vi "FolderMon Archive TDMS.vi"() -> ()   [LabVIEW 2011]
uses:
  <vilib>/Utility/miscctls.llb/LVDateTimeRec.ctl
  DIAdem/lib/DIAdem Daemon Queue.ctl
  DIAdem/lib/DIAdem Daemon Script Type.ctl
  ITK EXT/utils/strutil.llb/Case Matching.ctl
  server lib/Spartan Version.vi
  server lib/Spartan CONFIG Global.vi
  Summitek EXT/OpenG EXT/file/file.llb/File Exists - Scalar__ogtk.vi
  Summitek EXT/OpenG EXT/file/file.llb/Convert File Extension (Path)__ogtk.vi
panel:
  out "Files Archived":i32
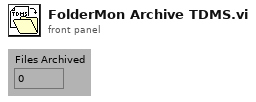
[diagram p1: front panel]
types:
  T1 = typedef "LVDateTimeRec.ctl" = cluster{"fractional second":dbl, "second":i32, "minute":i32, "hour":i32, "day of month":i32, "month":i32, "year":i32, "day of week":i32, "day of year":i32, "DST":i32}
  T2 = typedef "DIAdem Daemon Queue.ctl" = cluster{"Report Template TDM":path, "Report Processor VBS":path, "Report Path PDF":path, "Report Script Params":string, "Username":string, "Script Type":T3, "Report Query Params":string, "Client Machine":string, "Print on Client?":bool, "Response Queue Name":string, "Script Variables":string[], "Start Request Time":timestamp, "Wait?":bool}
  T3 = typedef "DIAdem Daemon Script Type.ctl" = enum16{"Report", "Query", "Script", "Datasheet", "Append", "Restart", "Stop"}
  T4 = typedef "Case Matching.ctl" = enum16{"a != A", "a == A", "system"}
  T5 = typedef "Keyed Array.ctl" = cluster{"keys":string[], "values":string[]}
  T6 = enum16{"open", "open or create", "create or replace", "create", "open (read-only)"}
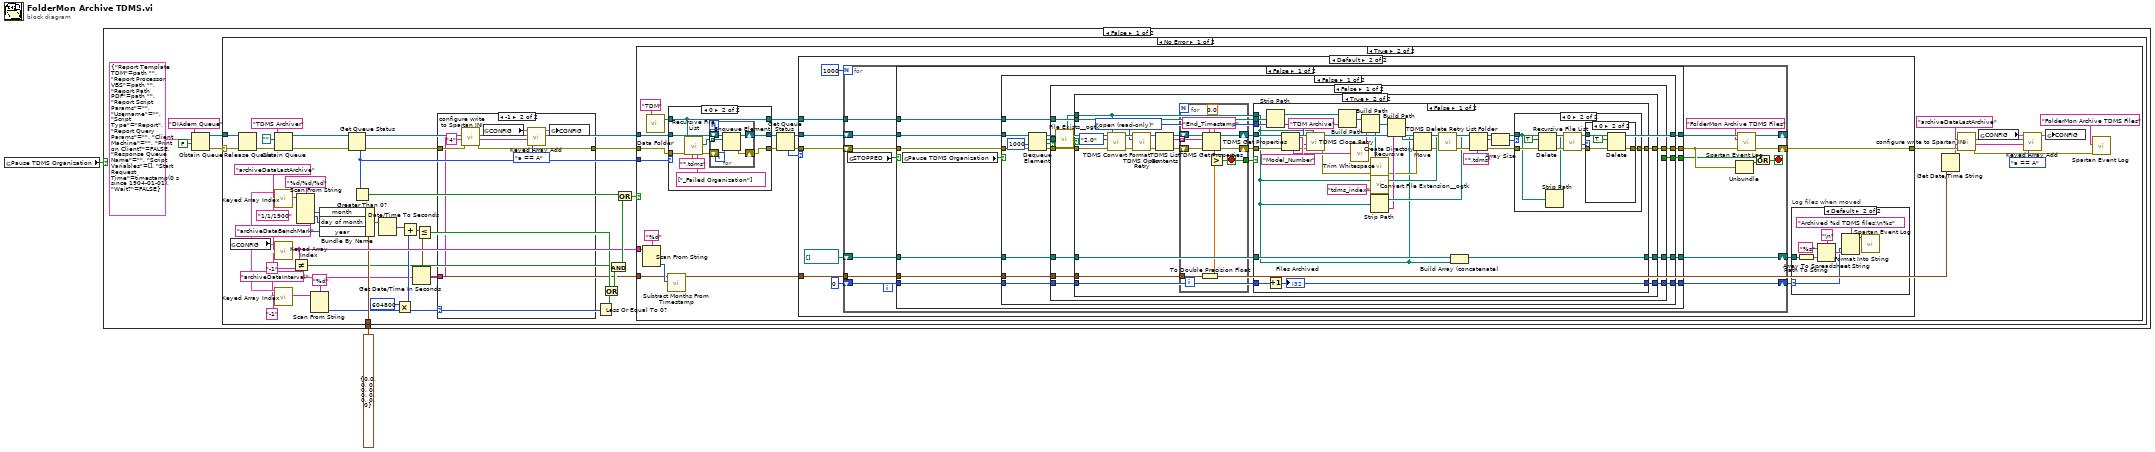
[diagram p0: block diagram]
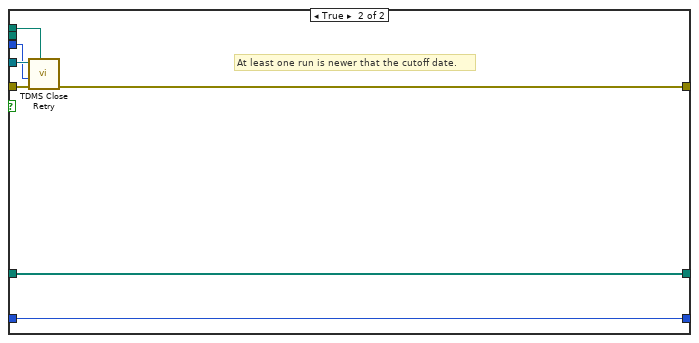
[diagram p9: hidden frame]
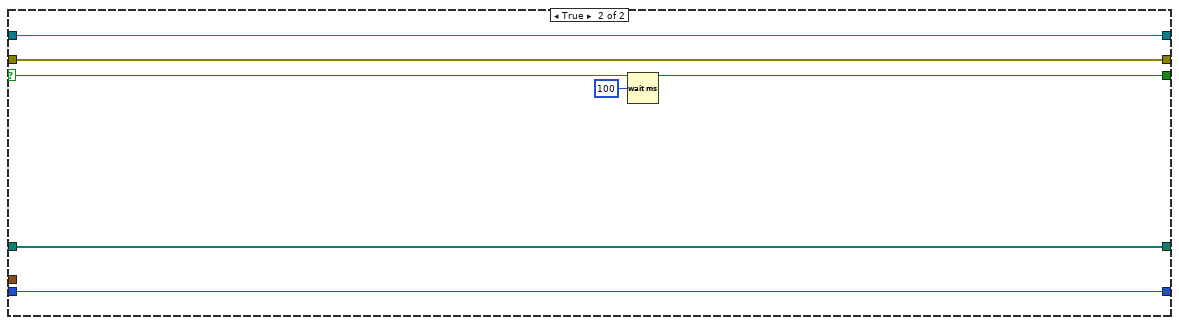
[diagram p11: hidden frame]
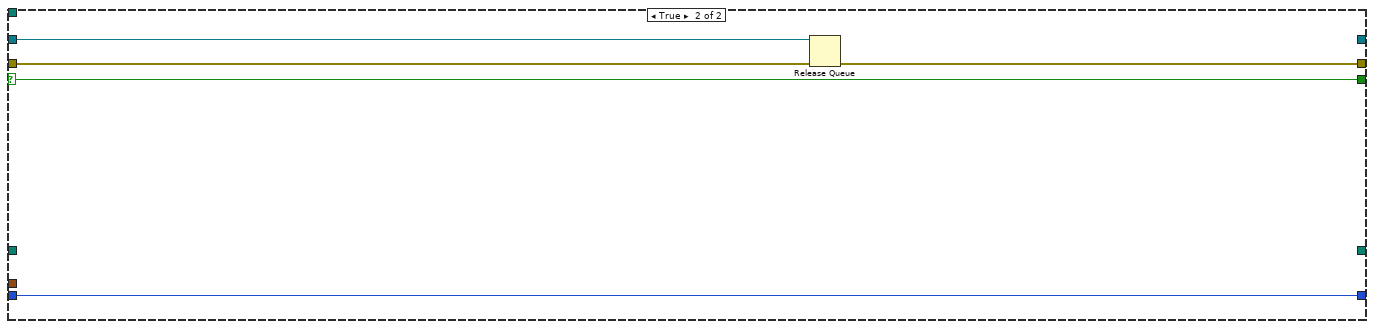
[diagram p12: hidden frame]
diagram:
  n1 = global read "Spartan Version.vi" "Pause TDMS Organization"() -> (w2:bool)
  n2 = case shown="False" w2 {
    tunnel: T1 {"fractional second"=0.0, "second"=0, "minute"=0, "hour"=0, "day of month"=0, "month"=0, "year"=0, "day of week"=0, "day of year"=0, "DST"=0} ("date time rec") -> [w3 _]
    frame False {
      n3 = Obtain Queue(name (unnamed)="DIAdem Queue", element data type=T2 {"Report Template TDM"=path "", "Report Processor VBS"=path "", "Report Path PDF"=path "", "Report Script Params"="", "Username"="", "Script Type"=enum."Report", "Report Query Params"="", "Client Machine"="", "Print on Client?"=FALSE, "Response Queue Name"="", "Script Variables"=[], "Start Request Time"=timestamp(0 s since 1904-01-01), "Wait?"=FALSE} ("DD_Report"), create if not found? (T)=FALSE) -> (queue out=w5:refnum<queue>, error out=w6:errorcluster)  [unwired: 2 in, 1 out]
      n4 = case shown="No Error" w6 {
        selector: w6 -> [w47 _]
        tunnel: w5 -> [w45 _]
        tunnel: w3 -> [w28 _]
        frame No Error {
          w14 = "archiveDataInterval"
          w43 = "-1" ("default value")
          n5 = global read "Spartan CONFIG Global.vi" "CONFIG"() -> (w29:T5)
          n6 = Release Queue(queue=w45, error in (no error)=w47) -> (error out=w46:errorcluster)  [unwired: 1 in, 2 out]
          n7 = Obtain Queue(name (unnamed)="TDMS Archiver", element data type=path "", error in (no error)=w46) -> (queue out=w37:refnum<queue>, error out=w36:errorcluster)  [unwired: 2 in, 1 out]
          n8 = call "Keyed Array Index.vi"("default value"="1/1/1900", "key"="archiveDataLastArchive", "array in"=w29) -> ("value"=w39:string)  [unwired: 1 in, 3 out]
          n9 = call "Keyed Array Index.vi"("default value"=w43, "key"="archiveDataBenchMark", "array in"=w29) -> ("value"=w32:string)  [unwired: 1 in, 3 out]
          n10 = call "Keyed Array Index.vi"("default value"="-1", "key"=w14, "array in"=w29) -> ("value"=w20:string)  [unwired: 1 in, 3 out]
          n11 = Not Equal?(x=w32, y=w43) -> (x != y?=w11:bool)
          n12 = Scan From String(format string="%d/%d/%d", input string=w39) -> (output 1=w27:i32, output 2=w26:i32, output 3=w25:i32)  [unwired: 5 in, 3 out]
          n13 = Scan From String(format string="%d", input string=w20) -> (output 1=w17:i32)  [unwired: 3 in, 3 out]
          n14 = Bundle By Name(cluster=w28, "month"=w27, "day of month"=w26, "year"=w25) -> (w24:T1)
          n15 = Get Queue Status(queue=w37, error in (no error)=w36) -> (queue out=w35:refnum<queue>, error out=w16:errorcluster, # elements in queue=w31:i32)  [unwired: 1 in, 5 out]
          n16 = Greater Than 0?(x=w31) -> (x > 0?=w34:bool)
          n17 = Date/Time To Seconds(2:w24) -> (0:w23:timestamp)  [unwired: 1 in]
          n18 = Multiply(x=604800, y=w17) -> (x*y=w22:i32)
          n19 = Add(x=w23, y=w22) -> (x+y=w18:timestamp)
          n20 = Get Date/Time In Seconds() -> (seconds since 1Jan1904=w9:timestamp)
          n21 = Less Or Equal?(x=w18, y=w9) -> (x <= y?=w13:bool)
          n22 = case shown="-1" w17 {
            tunnel: w16 -> [w50 w53]
            tunnel: [w50 w52] -> w15
            tunnel: w14 -> [_ w51]
            frame Default {
            }
            frame -1 {
              w57 = "4" ("Value (\"\")")
              n23 = call "configure write to Spartan INI.vi"("error in (no error)"=w53, "Value (\"\")"=w57, "Key (\"\")"=w51) -> ("error out"=w52:errorcluster)  [unwired: 8 in]
              n24 = global read "Spartan CONFIG Global.vi" "CONFIG"() -> (w55:T5)
              n25 = call "Keyed Array Add.vi"("case matching (sensitive)"=Case_Matching."a == A", "value"=w57, "key"=w51, "array in"=w55) -> ("array out"=w56:T5)  [unwired: 3 out]
              n26 = global write "Spartan CONFIG Global.vi" "CONFIG"(w56) -> ()
            }
          }
          n27 = Less Or Equal To 0?(x=w17) -> (x <= 0?=w12:bool)
          n28 = Or(x=w13, y=w12) -> (x .or. y?=w10:bool)
          n29 = And(x=w11, y=w10) -> (x .and. y?=w38:bool)
          n30 = Or(x=w34, y=w38) -> (x .or. y?=w33:bool)
          n31 = case shown="True" w33 {
            tunnel: w35 -> [_ w68]
            tunnel: w15 -> [_ w67]
            tunnel: w32 -> [_ w70]
            tunnel: w31 -> [_ w69]
            tunnel: w9 -> [_ w59]
            frame False {
            }
            frame True {
              w61 = "archiveDataLastArchive"
              n32 = Scan From String(format string="%d", input string=w70) -> (output 1=w72:i32)  [unwired: 3 in, 3 out]
              n33 = call "Data Folder.vi"("Relative Path (\"\" - Folder)"="TDM" ("Relative Path (\"\" - Folder)")) -> ("Data Folder"=w78:path)  [unwired: 2 in]
              n34 = call "Subtract Months From Timestamp.vi"("Months"=w72, "Start Time"=w59) -> ("End Time"=w71:timestamp)  [unwired: 9 in]
              n35 = case shown="0" w69 {
                tunnel: w68 -> [w82 w92]
                tunnel: [w84 w87] -> w77
                tunnel: w78 -> [w84 w87]
                tunnel: [w83 w89] -> w79
                tunnel: w67 -> [w83 w93]
                tunnel: [w82 w91] -> w80
                frame Default {
                }
                frame 0 {
                  n36 = call <vilib>:"Recursive File List.vi"("Folders to Exclude"=string[] ["_Failed Organization"], "pattern"="*.tdms", "error in (no error)"=w93, "Folder Path"=w87) -> ("error out"=w90:errorcluster, "All Files in Dir"=w86:path[])  [unwired: 3 in, 3 out]
                  n37 = for {
                    shift-right: [w97] -> w89
                    shift-left: w90 -> [w98]
                    tunnel: w86 -> [w95] mode=indexing
                    shift-right: [w94] -> w91
                    shift-left: w92 -> [w96]
                    n38 = Enqueue Element(queue=w96, element=w95, error in (no error)=w98) -> (queue out=w94:refnum<queue>, error out=w97:errorcluster)  [unwired: 1 in, 1 out]
                  }
                }
              }
              n39 = Get Queue Status(queue=w80, error in (no error)=w79) -> (queue out=w76:refnum<queue>, error out=w75:errorcluster, # elements in queue=w74:i32)  [unwired: 1 in, 5 out]
              n40 = case shown="Default" w74 {
                tunnel: w76 -> [_ w107]
                tunnel: w77 -> [_ w108]
                tunnel: w75 -> [w99 w106]
                tunnel: w71 -> [_ w103]
                tunnel: [w99 w100] -> w63
                frame 0 {
                }
                frame Default {
                  n41 = for {
                    N: 1000 -> [_]
                    tunnel: w108 -> [w122]
                    shift-right: [w115] -> w100
                    shift-left: w106 -> [w125]
                    shift-right: [w123] -> _
                    shift-left: w107 -> [w124]
                    shift-right: [w121] -> w101
                    shift-left: path[] [] -> [w118]
                    shift-right: [w117] -> w102
                    shift-left: 0 -> [w116]
                    tunnel: w103 -> [w114]
                    stop <- w120 stop-if-true
                    n42 = global read "Spartan Version.vi" "STOPPED"() -> (w110:bool)
                    n43 = case shown="False" w110 {
                      selector: w110 -> [_ w262]
                      tunnel: w125 -> [w134 w266]
                      tunnel: w124 -> [w133 w264]
                      tunnel: [w132 _] -> w123
                      tunnel: w122 -> [w137 _]
                      tunnel: [w136 w265] -> w112
                      tunnel: [w135 _] -> w121
                      tunnel: w118 -> [w131 _]
                      tunnel: [w130 w263] -> w117
                      tunnel: w116 -> [w129 w263]
                      tunnel: w114 -> [w127 _]
                      tunnel: [w126 w262] -> w111
                      frame False {
                        n44 = global read "Spartan Version.vi" "Pause TDMS Organization"() -> (w128:bool)
                        n45 = case shown="False" w128 {
                          selector: w128 -> [_ w256]
                          tunnel: w137 -> [w152 _]
                          tunnel: [w151 w261] -> w136
                          tunnel: [w150 w258] -> w135
                          tunnel: w134 -> [w149 w261]
                          tunnel: w133 -> [w147 w260]
                          tunnel: [w146 w260] -> w132
                          tunnel: w131 -> [w142 w258]
                          tunnel: [w141 w259] -> w130
                          tunnel: w129 -> [w140 w259]
                          tunnel: w127 -> [w139 _]
                          tunnel: [w138 w256] -> w126
                          frame False {
                            n46 = Dequeue Element(queue=w147, timeout in ms (-1)=1000, error in (no error)=w149) -> (queue out=w146:refnum<queue>, element=w145:path, timed out?=w143:bool, error out=w148:errorcluster)
                            n47 = case shown="False" w143 {
                              selector: w143 -> [_ w253]
                              tunnel: w152 -> [w162 _]
                              tunnel: [w161 w255] -> w151
                              tunnel: [w158 _] -> w150
                              tunnel: w148 -> [w160 w255]
                              tunnel: w145 -> [w153 _]
                              tunnel: w142 -> [w159 _]
                              tunnel: [w157 w254] -> w141
                              tunnel: w140 -> [w154 w254]
                              tunnel: w139 -> [w155 _]
                              tunnel: [_ w253] -> w138
                              frame False {
                                n48 = call-poly "File Exists__ogtk.vi"("file path"=w153) -> ("exists"=w156:bool)  [unwired: 6 in, 1 out]
                                n49 = case shown="True" w156 {
                                tunnel: w162 -> [_ w170]
                                tunnel: [w165 w172] -> w161
                                tunnel: w160 -> [w165 w185]
                                tunnel: w159 -> [w164 w169]
                                tunnel: [w164 w168] -> w158
                                tunnel: [w163 w166] -> w157
                                tunnel: w153 -> [_ w173]
                                tunnel: w155 -> [_ w177]
                                tunnel: w154 -> [w163 w167]
                                frame False {
                                }
                                frame True {
                                w174 = T6."open (read-only)" ("operation (0:open)")
                                n50 = call <vilib>:"TDMS Convert Format.vi"("error in (no error)"=w185, "target version"=enum16{"1.0", "2.0"}."2.0", "file path"=w173) -> ("error out"=w184:errorcluster, "file path out"=w183:path)  [unwired: 3 in]
                                n51 = call "TDMS Open Retry.vi"("error in (no error)"=w184, "Operation (0:open)"=w174, "Path"=w183) -> ("error out"=w181:errorcluster, "TDMS File Ref"=w182:refnum<k34>)  [unwired: 1 in, 6 out]
                                n52 = TDMS List Contents(4:w181, 7:w182) -> (0:w180:errorcluster, 2:w178:string[], 3:w179:refnum<k34>)  [unwired: 1 in, 1 out]
                                n53 = for {
                                shift-right: [w243] -> w175
                                shift-left: w180 -> [w252]
                                shift-right: [w242] -> w176
                                shift-left: w179 -> [w251]
                                tunnel: w178 -> [w250] mode=indexing
                                tunnel: w177 -> [w246]
                                tunnel: [w244] -> w171
                                stop <- w244 stop-if-true
                                n54 = To Double Precision Float(number=w246) -> (double precision float=w245:dbl)
                                n55 = TDMS Get Properties(5:0.0, 7:"End_Timestamp" ("property name"), 8:w252, 10:w250, 11:w251) -> (0:w243:errorcluster, 3:w242:refnum<k34>, 4:w247:dbl)  [unwired: 1 in, 3 out]
                                n56 = Greater?(x=w247, y=w245) -> (0:w244:bool)
                                }
                                n57 = case shown="False" w171 {
                                tunnel: w176 -> [w218 w241]
                                tunnel: w175 -> [w219 w240]
                                tunnel: w174 -> [w209 w239]
                                tunnel: w173 -> [w187 w235]
                                tunnel: [w200 w238] -> w172
                                tunnel: w170 -> [w217 _]
                                tunnel: w169 -> [w198 w236]
                                tunnel: [w197 w236] -> w168
                                tunnel: w167 -> [w196 w237]
                                tunnel: [w195 w237] -> w166
                                frame False {
                                w211 = "Model_Number" ("Property Name")
                                n58 = Strip Path(path=w217) -> (stripped path=w216:path)  [unwired: 1 out]
                                n59 = Increment(x=w196) -> (x+1=w195:i32)
                                "Files Archived" <- w195
                                n60 = TDMS Get Properties(5:w211, 7:w211, 8:w219, 11:w218) -> (0:w192:errorcluster, 3:w208:refnum<k34>, 4:w210:string)  [unwired: 2 in, 3 out]
                                n61 = call "TDMS Close Retry.vi"("TDMS Path"=w187, "error in (no error)"=w192, "Operation (0:open)"=w209, "TDMS File Ref"=w208) -> ("error out"=w191:errorcluster)  [unwired: 5 in, 2 out]
                                n62 = Build Path(base path=w216, name or relative path="TDM Archive") -> (appended path=w213:path)
                                n63 = call <vilib>:"Trim Whitespace.vi"("string"=w210) -> ("trimmed string"=w214:string)  [unwired: 1 in]
                                n64 = Build Path(base path=w213, name or relative path=w214) -> (appended path=w212:path)
                                n65 = call <vilib>:"Create Directory Recursive.vi"("error in (no error)"=w191, "directory"=w212) -> ("error out"=w188:errorcluster)  [unwired: 1 in, 4 out]
                                n66 = call-poly "Convert File Extension__ogtk.vi"("new ending (none)"="tdms_index", "file name"=w187) -> ("new filename"=w206:path)  [unwired: 1 out]
                                n67 = Strip Path(path=w187) -> (stripped path=w199:path, name=w193:string)
                                n68 = Build Path(base path=w212, name or relative path=w193) -> (appended path=w190:path)
                                n69 = Move(source path=w187, error in=w188, 10:w190) -> (error out=w189:errorcluster)  [unwired: 2 in, 2 out]
                                n70 = call "TDMS Delete Retry.vi"("error in"=w189, "path (use dialog)"=w206) -> ("error out"=w205:errorcluster)  [unwired: 9 out]
                                n71 = Build Array (concatenate)(w198, w187) -> (w197:path[])
                                n72 = List Folder(path=w199, pattern="*.tdms", error in=w205) -> (path out=w194:path, filenames=w203:string[], error out=w201:errorcluster)  [unwired: 1 in, 1 out]
                                n73 = Array Size(array=w203) -> (size(s)=w202:i32)
                                n74 = case shown="0" w202 {
                                tunnel: w201 -> [w220 w229]
                                tunnel: [w220 w225] -> w200
                                tunnel: w194 -> [_ w221]
                                frame Default {
                                }
                                frame 0 {
                                n75 = Delete(path (use dialog)=w221, entire hierarchy (F)=TRUE, error in=w229) -> (error out=w227:errorcluster)  [unwired: 2 in, 2 out]
                                n76 = Strip Path(path=w221) -> (stripped path=w224:path)  [unwired: 1 out]
                                n77 = call <vilib>:"Recursive File List.vi"("error in (no error)"=w227, "Folder Path"=w224) -> ("error out"=w226:errorcluster, "Number of Files"=w223:i32, "dup Folder Path"=w222:path)  [unwired: 5 in, 2 out]
                                n78 = case shown="0" w223 {
                                tunnel: w226 -> [w230 w233]
                                tunnel: [w230 w232] -> w225
                                tunnel: w222 -> [_ w231]
                                frame Default {
                                }
                                frame 0 {
                                n79 = Delete(path (use dialog)=w231, entire hierarchy (F)=TRUE, error in=w233) -> (error out=w232:errorcluster)  [unwired: 2 in, 2 out]
                                }
                                }
                                }
                                }
                                }
                                frame True {
                                # "At least one run is newer that the cutoff date."
                                n80 = call "TDMS Close Retry.vi"("TDMS Path"=w235, "error in (no error)"=w240, "Operation (0:open)"=w239, "TDMS File Ref"=w241) -> ("error out"=w238:errorcluster)  [unwired: 5 in, 2 out]
                                }
                                }
                                }
                                }
                              }
                              frame True {
                              }
                            }
                          }
                          frame True {
                            n81 = Wait (ms)(milliseconds to wait=u32 100) -> ()  [unwired: 1 out]
                          }
                        }
                      }
                      frame True {
                        n82 = Release Queue(queue=w264, error in (no error)=w266) -> (error out=w265:errorcluster)  [unwired: 1 in, 2 out]
                      }
                    }
                    n83 = Unbundle(w112) -> ("status"=w119:bool)  [unwired: 2 out]
                    n84 = call "Spartan Event Log.vi"("error in (no error)"=w112, "module (\"\")"="FolderMon Archive TDMS Files" ("name (unnamed)")) -> ("error out"=w115:errorcluster)  [unwired: 3 in, 3 out]
                    n85 = Or(x=w111, y=w119) -> (x .or. y?=w120:bool)
                  }
                  n86 = case "Log files when moved" shown="Default" w102 {
                    selector: w102 -> [_ w267]
                    tunnel: w101 -> [_ w268]
                    frame 0 {
                    }
                    frame Default {
                      n87 = Path To String(path=w268) -> (string=w272:string[])
                      n88 = Array To Spreadsheet String(delimiter (Tab)="\n", array=w272, 3:"%s" ("delimiter (Tab)")) -> (spreadsheet string=w269:string)
                      n89 = Format Into String(format string="Archived %d TDMS files:\n%s" ("name (unnamed)"), w267, w269) -> (resulting string=w273:string)  [unwired: 2 in, 1 out]
                      n90 = call "Spartan Event Log.vi"("message (\"\")"=w273) -> ()  [unwired: 4 in, 4 out]
                    }
                  }
                }
              }
              n91 = Get Date/Time String(seconds (now)=w59) -> (date string=w58:string)  [unwired: 2 in, 1 out]
              n92 = call "configure write to Spartan INI.vi"("error in (no error)"=w63, "Value (\"\")"=w58, "Key (\"\")"=w61) -> ("error out"=w60:errorcluster)  [unwired: 8 in]
              n93 = global read "Spartan CONFIG Global.vi" "CONFIG"() -> (w65:T5)
              n94 = call "Keyed Array Add.vi"("case matching (sensitive)"=Case_Matching."a == A", "value"=w58, "key"=w61, "array in"=w65) -> ("array out"=w66:T5)  [unwired: 3 out]
              n95 = global write "Spartan CONFIG Global.vi" "CONFIG"(w66) -> ()
              n96 = call "Spartan Event Log.vi"("error in (no error)"=w60, "module (\"\")"="FolderMon Archive TDMS Files" ("name (unnamed)")) -> ()  [unwired: 3 in, 4 out]
            }
          }
        }
        frame Error {
        }
      }
    }
    frame True {
    }
  }
